vi "ChangeRightSubpanel.vi"(8 "error in (no error)":errorcluster, 10 "Left Active":i32, 11 "MAUI in":refnum<class "MAUI.lvclass">) -> (0 "error out":errorcluster, 3 "MAUI out":refnum<class "MAUI.lvclass">)   [LabVIEW 2016, in "MAUI.lvclass"]
uses:
  MAUI.lvclass
  MAUI.lvclass/MAUI.ctl
  <vilib>/Levylab/Embedded SMO UI/EmbeddedSMO.lvclass
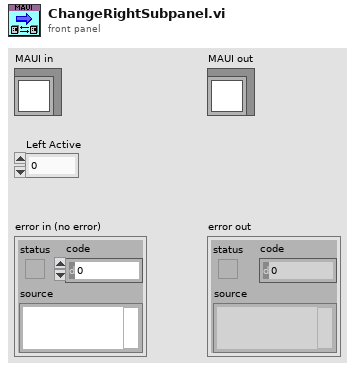
[diagram p1: front panel]
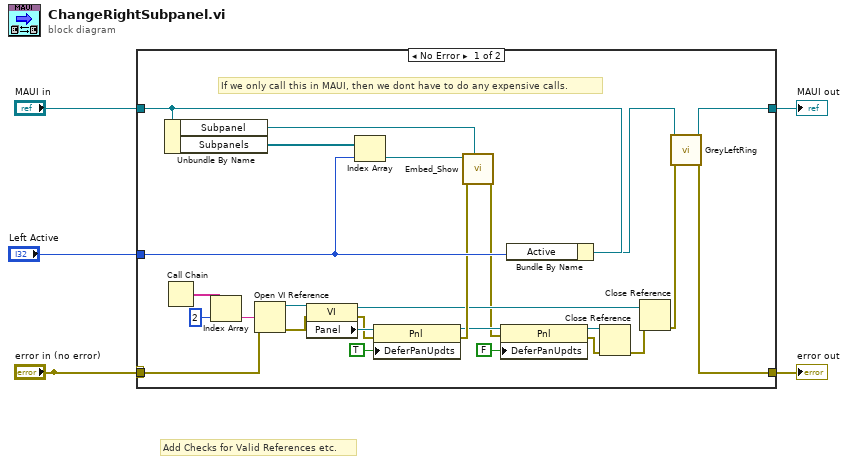
[diagram p0: block diagram]
diagram:
  # "Add Checks for Valid References etc."
  n1 = case shown="No Error" "error in (no error)" {
    selector: "error in (no error)" -> [_ w33]
    tunnel: [w24 w33] -> w5
    tunnel: [w25 w32] -> w3
    tunnel: "MAUI in" -> [w27 w32]
    tunnel: "Left Active" -> [w31 _]
    tunnel: "error in (no error)" -> [w20 _]
    frame No Error {
      # "If we only call this in MAUI, then we dont have to do any expensive calls."
      n2 = Unbundle By Name(w27) -> ("Subpanel"=w30:refnum<vi>, "Subpanels"=w29:refnum<class "EmbeddedSMO.lvclass">[])
      n3 = Call Chain() -> (call chain=w23:string[])
      n4 = Index Array(array=w23, index=2) -> (element=w21:string)
      n5 = Open VI Reference(vi path=w21, error in (no error)=w20) -> (vi reference=w19:refnum<vi>, error out=w15:errorcluster)  [unwired: 4 in]
      n6 = property class="VI"(reference=w19, error in=w15) -> (reference out=w13:refnum<vi>, error out=w16:errorcluster, "Panel"=w18:refnum<vi>)
      n7 = Index Array(array=w29, index=w31) -> (element=w28:refnum<class "EmbeddedSMO.lvclass">)
      n8 = property class="Pnl"(reference=w18, error in=w16, "DeferPanUpdts"=TRUE ("Defer Panel Updates")) -> (reference out=w12:refnum<vi>, error out=w14:errorcluster)
      n9 = call <vilib>:"Embed_Show.vi"("Sub Panel"=w30, "error in (no error)"=w14, "EmbeddedSMO in"=w28) -> ("error out"=w7:errorcluster)  [unwired: 7 in, 1 out]
      n10 = property class="Pnl"(reference=w12, error in=w7, "DeferPanUpdts"=FALSE ("Defer Panel Updates")) -> (reference out=w10:refnum<vi>, error out=w9:errorcluster)
      n11 = Bundle By Name(cluster=w27, "Active"=w31) -> (w26:refnum<class "MAUI.lvclass">)
      n12 = Close Reference(reference=w10, error in (no error)=w9) -> (error out=w8:errorcluster)
      n13 = Close Reference(reference=w13, error in (no error)=w8) -> (error out=w6:errorcluster)
      n14 = call "GreyLeftRing.vi"("error in (no error)"=w6, "MAUI in"=w26) -> ("error out"=w24:errorcluster, "MAUI out"=w25:refnum<class "MAUI.lvclass">)  [unwired: 8 in]
    }
    frame Error {
    }
  }
  "error out" <- w5
  "MAUI out" <- w3
